vi "2D Auto Correlation (CDB).vi"(11 "X":cdb[][](array[numeric])) -> (0 "error":i32, 3 "Rxx":cdb[][](array[numeric]))   [LabVIEW 2018, in "NI_AALPro.lvlib"]
doc: "Computes the autocorrelation of the input sequence <B>X</B>. Wire data to the <B>X</B> input to determine the polymorphic instance to use or manually select the instance."
uses:
  NI_AALPro.lvlib
  <resource>/lvanlys.dll
panel:
  # "2D AutoCorrelation (CDB)"
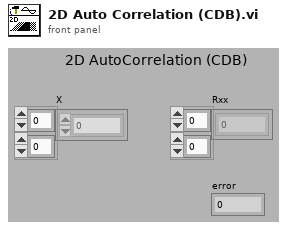
[diagram p1: front panel]
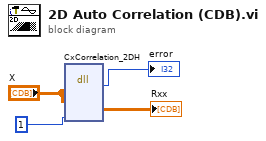
[diagram p0: block diagram]
diagram:
  n1 = dll-call lib="C:/Program Files (x86)/National Instruments/LabVIEW 2018/resource/lvanlys.*" fn="CxCorrelation_2DH"("X"="X", "X"="X", "domain"=1 ("conv_corr")) -> (→"error":i32, "Rxx"=→"Rxx":cdb[][])  [unwired: 7 in, 2 out]
